vi "FRC Simulated.vi"() -> ()   [LabVIEW 2015]
doc: "This VI starts and stops the environment simulator and serves as the master VI for your simulation code. Open and run this VI to display the environment simulator, or open the block diagram to view or modify simulation code."
uses:
  <vilib>/Rock Robotics/SystemInterfaces/DIO/FPGA_DIOPWMChannel.ctl
  <vilib>/Rock Robotics/WPI/MotorControl/WPI_MotorControlOpen VictorSP.vi
  <vilib>/Rock Robotics/WPI/RobotDrive/WPI_RobotDriveOpen2MotorWithVictorSP.vi
  <vilib>/robotics/Simulator/NI_Robotics_Simulator.lvlib
panel:
  in  "Right Drive Motors":dbl(slide) scale=-1.0..1.0
  in  "Left Drive Motors":dbl(slide) scale=-1.0..1.0
  in  "Arm Pivot":dbl(slide) scale=-1.0..1.0
  in  "Arm Angle":dbl(knob)
  in  "manifest filename":string="FRC Simulated.xml"
  in  "stop":bool
  # "* Press the Run button to display the Robotics Environment Simulator.\n* Select Window>>Show Block Diagram or press <Ctrl-E> to view the block diagram, where you can add or modify simulation code. Add controls and indicators to the front panel of this VI to pass data into and out of the simulation code.\n* The manifest file must exist in same directory as the .lvproj file."
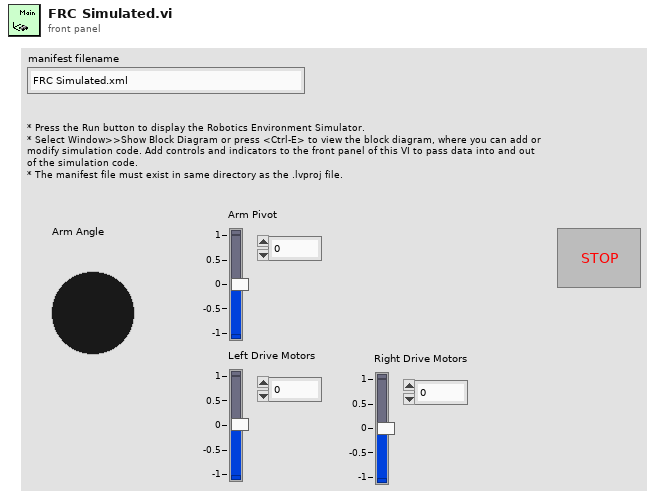
[diagram p1: front panel]
types:
  T1 = typedef "FPGA_DIOPWMChannel.ctl" = enum8{"PWM 0", "PWM 1", "PWM 2", "PWM 3", "PWM 4", "PWM 5", "PWM 6", "PWM 7", "PWM 8", "PWM 9", "PWM MXP 0", "PWM MXP 1", "PWM MXP 2", "PWM MXP 3", "PWM MXP 4", "PWM MXP 5", "PWM MXP 6", "PWM MXP 7", "PWM MXP 8", "PWM MXP 9", "Invalid"}
  T2 = typedef "WPI_ServoDeviceRef.ctl" = cluster{"DeviceStatus":errorcluster, "PWM Channel":T1, "DeadBand":T3}
  T3 = typedef "WPI_PWMDeadband.ctl" = cluster{"Name":string, "maxPositivePwm":i32, "minPositivePwm":i32, "centerPwm":i32, "maxNegativePwm":i32, "minNegativePwm":i32, "angularRange":u16}
  T4 = typedef "WPI_RobotDriveDevRef.ctl" = cluster{"DevStatus":errorcluster, "Motors[]":T5[], "Square Inputs":bool, "Max Output":dbl}
  T5 = typedef "WPI_MotorControlDeviceRef.ctl" = cluster{"DeviceStatus":errorcluster, "Type":T6, "PWM":cluster{"PWM Channel":T1, "DeadBand":T3}, "CAN":cluster{"Device Number":u8, "Control Mode":T7, "Semaphore":T8, "Max Vout":dbl, "TalonSRX Control Mode":T9}, "Invert":bool}
  T6 = typedef "WPI_MotorControlType.ctl" = enum16{"PWM", "CAN", "CANTalonSRX"}
  T7 = typedef "WPI_CANJaguar_ControlMode.ctl" = enum8{"Percent VBus", "Current", "Speed", "Position", "Voltage"}
  T8 = typedef "Semaphore RefNum" = refnum<k1>
  T9 = typedef "WPI_CANTalonSRX_APIControlMode.ctl" = enum8{"Percent VBus", "Speed", "Position", "Slave", "Unchanged / Invalid", "Voltage Compensation", "Current", "Motion Profile"}
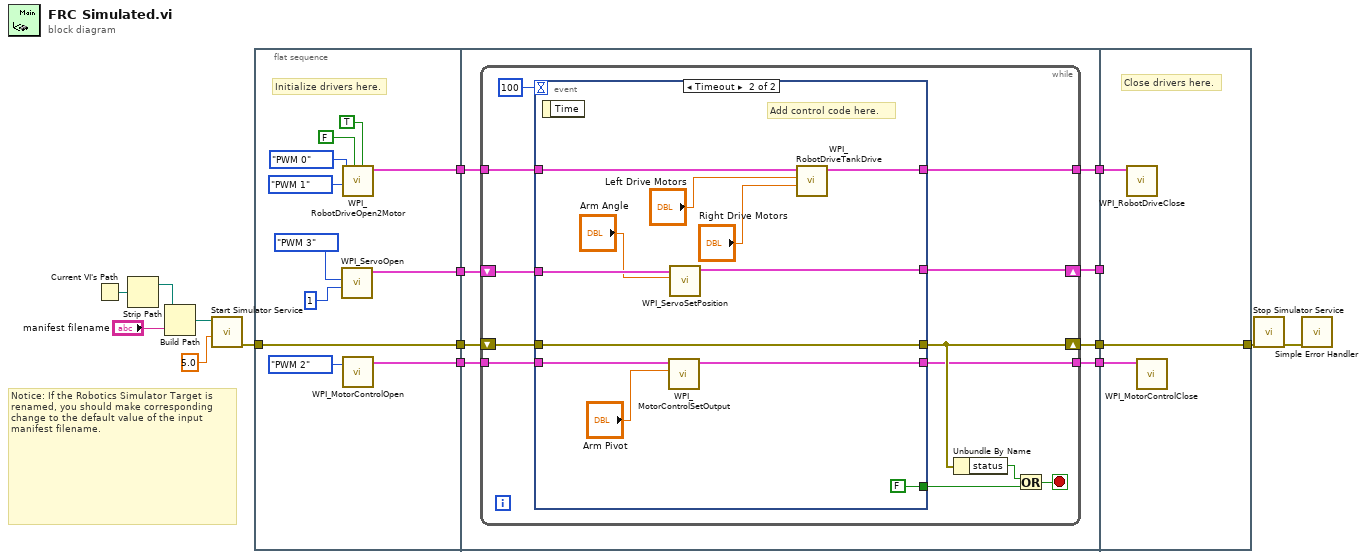
[diagram p0: block diagram]
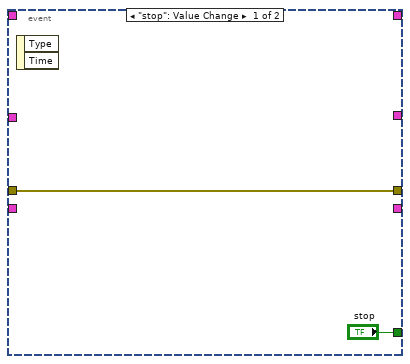
[diagram p2: hidden frame]
diagram:
  # "Notice: If the Robotics Simulator Target is renamed, you should make corresponding change to the default value of the input manifest filename."
  n1 = Current VI's Path() -> (path=w14:path)
  n2 = Strip Path(path=w14) -> (stripped path=w13:path)  [unwired: 1 out]
  n3 = Build Path(base path=w13, name or relative path="manifest filename") -> (appended path=w12:path)
  n4 = call <vilib>:"Start Simulator Service.vi"("step size (ms)"=5.0 ("stepsize(ms)"), "manifest file"=w12) -> ("error out"=w9:errorcluster)  [unwired: 9 in]
  n5 = flat-sequence {
    tunnel: w9 -> [w27]
    tunnel: [w27] -> w8
    tunnel: [w25] -> w6
    tunnel: [w22] -> w4
    tunnel: [w17] -> w2
    tunnel: w8 -> [w34]
    tunnel: [w35] -> w7
    tunnel: w6 -> [w33]
    tunnel: [w32] -> w5
    tunnel: w4 -> [w31]
    tunnel: [w30] -> w3
    tunnel: w2 -> [w29]
    tunnel: [w28] -> w1
    tunnel: [w64] -> w15
    tunnel: w7 -> [w64]
    tunnel: w5 -> [_]
    tunnel: w3 -> [w63]
    tunnel: w1 -> [w62]
    frame #0 {
      # "Initialize drivers here."
      n6 = call <vilib>:"WPI_ServoOpen.vi"("Angular Range"=u16 1, "PWM Channel"=FPGA_DIOPWMChannel."PWM 3") -> ("ServoDeviceRef"=w25:T2)  [unwired: 8 in, 1 out]
      n7 = call-poly <vilib>:"WPI_RobotDriveOpen2Motor.vi"("Right Motor Inverted"=TRUE, "Left Motor Inverted"=FALSE, "Right Motor"=FPGA_DIOPWMChannel."PWM 1", "Left Motor"=FPGA_DIOPWMChannel."PWM 0") -> ("RobotDriveDevRef"=w17:T4)  [unwired: 6 in, 1 out]
      n8 = call-poly <vilib>:"WPI_MotorControlOpen.vi"("PWM Channel"=FPGA_DIOPWMChannel."PWM 2") -> ("MotorControlDeviceRef"=w22:T5)  [unwired: 9 in, 1 out]
    }
    frame #1 {
      n9 = while {
        shift-right: [w43] -> w35
        shift-left: w34 -> [w46]
        shift-right: [w40] -> w32
        shift-left: w33 -> [w41]
        tunnel: w31 -> [w39]
        tunnel: [w38] -> w30
        tunnel: w29 -> [w37]
        tunnel: [w36] -> w28
        stop <- w44 stop-if-true
        n10 = event shown="[1] Timeout" {
          selector: _ -> [_ _]
          dyn-events: _ -> [_ _]
          timeout: 100 -> [_ _]
          tunnel: ["stop" FALSE ("stop")] -> w45
          tunnel: [w48 w61] -> w43
          tunnel: w46 -> [w48 w61]
          tunnel: w41 -> [_ w59]
          tunnel: [_ w58] -> w40
          tunnel: w39 -> [_ w56]
          tunnel: [_ w54] -> w38
          tunnel: w37 -> [_ w53]
          tunnel: [_ w50] -> w36
          event "stop": Value Change {
            n11 = event-data() -> ()  [unwired: 1 in, 2 out]
          }
          event Timeout {
            # "Add control code here."
            n12 = event-data() -> ()  [unwired: 1 in, 1 out]
            n13 = call <vilib>:"WPI_MotorControlSetOutput.vi"("Output"="Arm Pivot", "MotorControlDevRef"=w56) -> ("MotorControlDevRef"=w54:T5)  [unwired: 7 in, 2 out]
            n14 = call <vilib>:"WPI_ServoSetPosition.vi"("Position"="Arm Angle", "ServoDeviceRef"=w59) -> ("ServoDeviceRef"=w58:T2)  [unwired: 8 in, 1 out]
            n15 = call <vilib>:"WPI_RobotDriveTankDrive.vi"("Right axis value"="Right Drive Motors", "Left axis value"="Left Drive Motors", "RobotDriveDevRef"=w53) -> ("RobotDriveDevRef"=w50:T4)  [unwired: 6 in, 2 out]
          }
        }
        n16 = Unbundle By Name(w43) -> ("status"=w42:bool)
        n17 = Or(x=w42, y=w45) -> (x .or. y?=w44:bool)
      }
    }
    frame #2 {
      # "Close drivers here."
      n18 = call <vilib>:"WPI_RobotDriveClose.vi"("RobotDriveDevRef"=w62) -> ()  [unwired: 10 in, 1 out]
      n19 = call <vilib>:"WPI_MotorControlClose.vi"("MotorControlDevRef"=w63) -> ()  [unwired: 10 in, 1 out]
    }
  }
  n20 = call <vilib>:"Stop Simulator Service.vi"("error in (no error)"=w15) -> ("error out"=w10:errorcluster)  [unwired: 10 in]
  n21 = call <vilib>:"Simple Error Handler.vi"("error in (no error)"=w10) -> ()  [unwired: 4 in, 5 out]
